vi "SETPINSTATUS.vi"(0 "NXP in":refnum<class "NXP.lvclass">, 5 "PORT":dbl, 7 "PIN":dbl, 9 "valor":bool, 11 "error in (no error)":errorcluster) -> (4 "NXP out":refnum<class "NXP.lvclass">, 15 "error out":errorcluster)   [LabVIEW 2019, in "NXP.lvclass"]
uses:
  NXP.lvclass
  NXP.lvclass/NXP.ctl
  2c465943-1315-438f-b26f-e32eb19f3964.vi
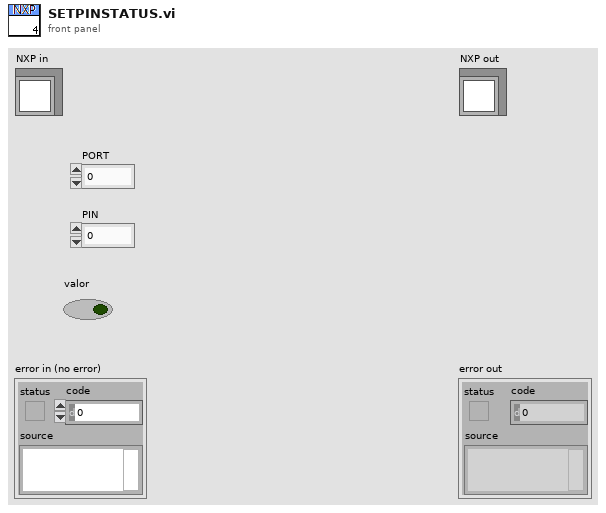
[diagram p1: front panel]
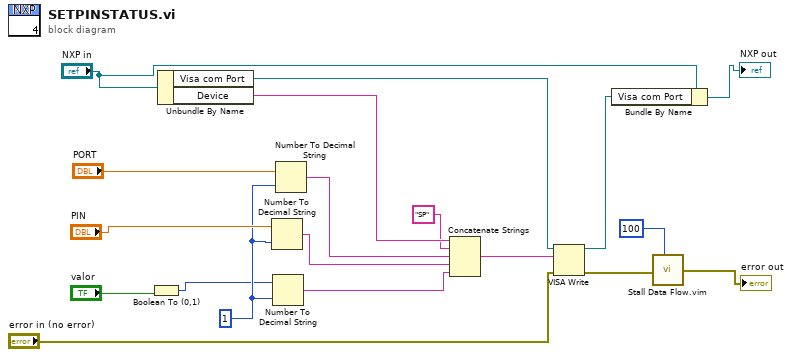
[diagram p0: block diagram]
diagram:
  w17 = i16 1 ("width (-)")
  n1 = Boolean To (0,1)(Boolean="valor") -> (0, 1=w15:i16)
  n2 = Unbundle By Name("NXP in") -> ("Visa com Port"=w8:refnum<visa-resource-name>, "Device"=w14:string)
  n3 = Number To Decimal String(number="PIN", width (-)=w17) -> (decimal integer string=w11:string)
  n4 = Number To Decimal String(number=w15, width (-)=w17) -> (decimal integer string=w10:string)
  n5 = Number To Decimal String(number="PORT", width (-)=w17) -> (decimal integer string=w12:string)
  n6 = Concatenate Strings(w14, "SP" ("string"), w12, w11, w10) -> (w9:string)
  n7 = VISA Write(VISA resource name=w8, write buffer=w9, error in (no error)="error in (no error)") -> (VISA resource name out=w1:refnum<visa-resource-name>, error out=w6:errorcluster)  [unwired: 1 out]
  n8 = Bundle By Name(cluster="NXP in", "Visa com Port"=w1) -> (→"NXP out":refnum<class "NXP.lvclass">)
  n9 = call "Stall Data Flow.vim"("value in"=w6, "milliseconds to wait"=u32 100) -> ("value out"=→"error out":errorcluster)  [unwired: 1 out]
